vi "Read Device Name.vi"(8 "Error In":errorcluster, 11 "object in":refnum<class "Instrument.lvclass">) -> (0 "Error Out":errorcluster, 2 "HW Device Name":string, 3 "object out":refnum<class "Instrument.lvclass">)   [LabVIEW 2023, in "HAL.lvlib" / "Instrument.lvclass"]
uses:
  Instrument.lvclass
  Instrument.lvclass/Instrument.ctl
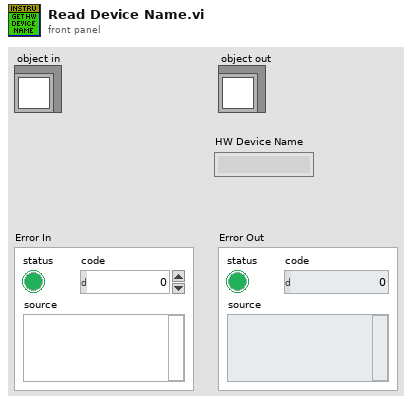
[diagram p1: front panel]
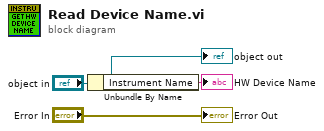
[diagram p0: block diagram]
diagram:
  n1 = Unbundle By Name("object in") -> ("Instrument Name"=→"HW Device Name":string)
  "Error Out" <- "Error In"
  "object out" <- "object in"
